vi "test-state-space-utils.vi"() -> ()   [LabVIEW 2019]
uses:
  <vilib>/Rock Robotics/WPI/ThirdParty/JAS_Junk/TrajLib/LINEAR_SYSTEM.ctl
  <vilib>/Analysis/Matrix/Datatypes/RealMatrix.ctl
  <vilib>/Rock Robotics/WPI/ThirdParty/JAS_Junk/TrajLib/LINEAR_QUADRATIC_REGULATOR.ctl
  <vilib>/Rock Robotics/WPI/ThirdParty/JAS_Junk/TrajLib/DCMotor_New.vi
  <vilib>/Rock Robotics/WPI/ThirdParty/JAS_Junk/TrajLib/Units_RotationsPerMinuteToRadiansPerSecond.vi
  <vilib>/Rock Robotics/WPI/ThirdParty/JAS_Junk/TrajLib/LinearSystem_New.vi
  <vilib>/Rock Robotics/WPI/ThirdParty/JAS_Junk/TrajLib/MatBuilder_Create.vi
  <vilib>/Rock Robotics/WPI/ThirdParty/JAS_Junk/TrajLib/MatBuilder_Fill.vi
  <vilib>/Rock Robotics/WPI/ThirdParty/JAS_Junk/TrajLib/MatrixHelper_Zero.vi
  <vilib>/Rock Robotics/WPI/ThirdParty/JAS_Junk/TrajLib/MatrixHelper_CoerceSize.vi
  <vilib>/Rock Robotics/WPI/ThirdParty/JAS_Junk/TrajLib/Trajectory_Library.lvlib
  <vilib>/Analysis/Matrix/NI_Matrix.lvlib
panel:
  out "LQR New Sys-ELMS Error":bool
  out "LQR New Error":bool
  out "LQR New":T1
  out "Rcost":T2
  out "Qcost":T2
  out "Relms":T2
  out "Qelms":T2
  out "LQR New Sys-ELMS":T1
  out "ElevatorSystem":T3
  # "Ref State <States,1>"
  # "Comp and capped \noutput <Inputs,1>"
  # "Controller gain\n<Inputs,States>"
  # "Ref State <States,1>"
  # "Comp and capped \noutput <Inputs,1>"
  # "Controller gain\n<Inputs,States>"
  # "<States,States>"
  # "<States,Inputs>"
  # "<Outputs,States>"
  # "<Outputs,Inputs>"
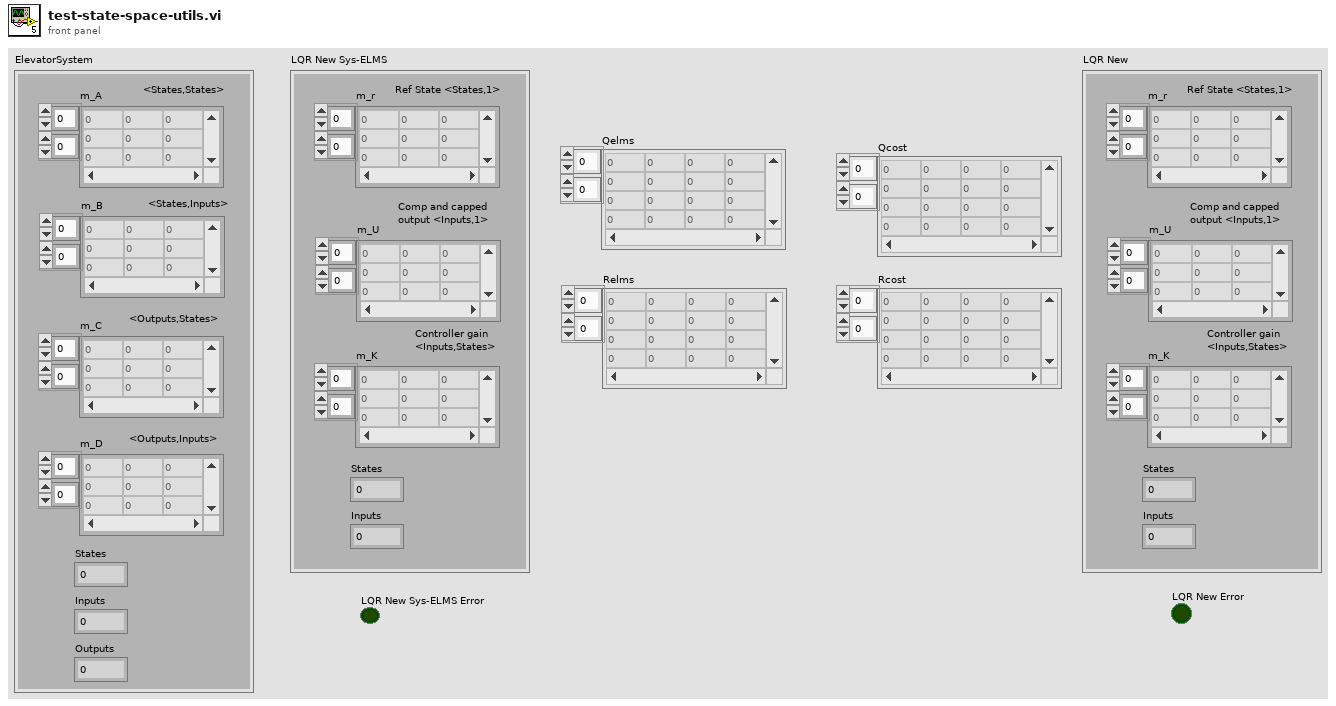
[diagram p1: front panel]
types:
  T1 = typedef "Trajectory_Library.lvlib/LINEAR_QUADRATIC_REGULATOR.ctl" = cluster{"m_r":T2, "m_U":T2, "m_K":T2, "States":i32, "Inputs":i32}
  T2 = typedef "NI_Matrix.lvlib/RealMatrix.ctl" = dbl[][]
  T3 = typedef "Trajectory_Library.lvlib/LINEAR_SYSTEM.ctl" = cluster{"m_A":T2, "m_B":T2, "m_C":T2, "m_D":T2, "States":i32, "Inputs":i32, "Outputs":i32}
  T4 = typedef "Trajectory_Library.lvlib/DCMOTOR.CTL" = cluster{"nominalVoltage_Volts":dbl, "StallTorque_NM":dbl, "StallCurrent_Amps":dbl, "FreeCurrent_Amps":dbl, "FreeSpeed_RadPerSec":dbl, "R_Ohms":dbl, "Kv_RadPerSecPerVolt":dbl, "Kt_NMPerAmp":dbl}
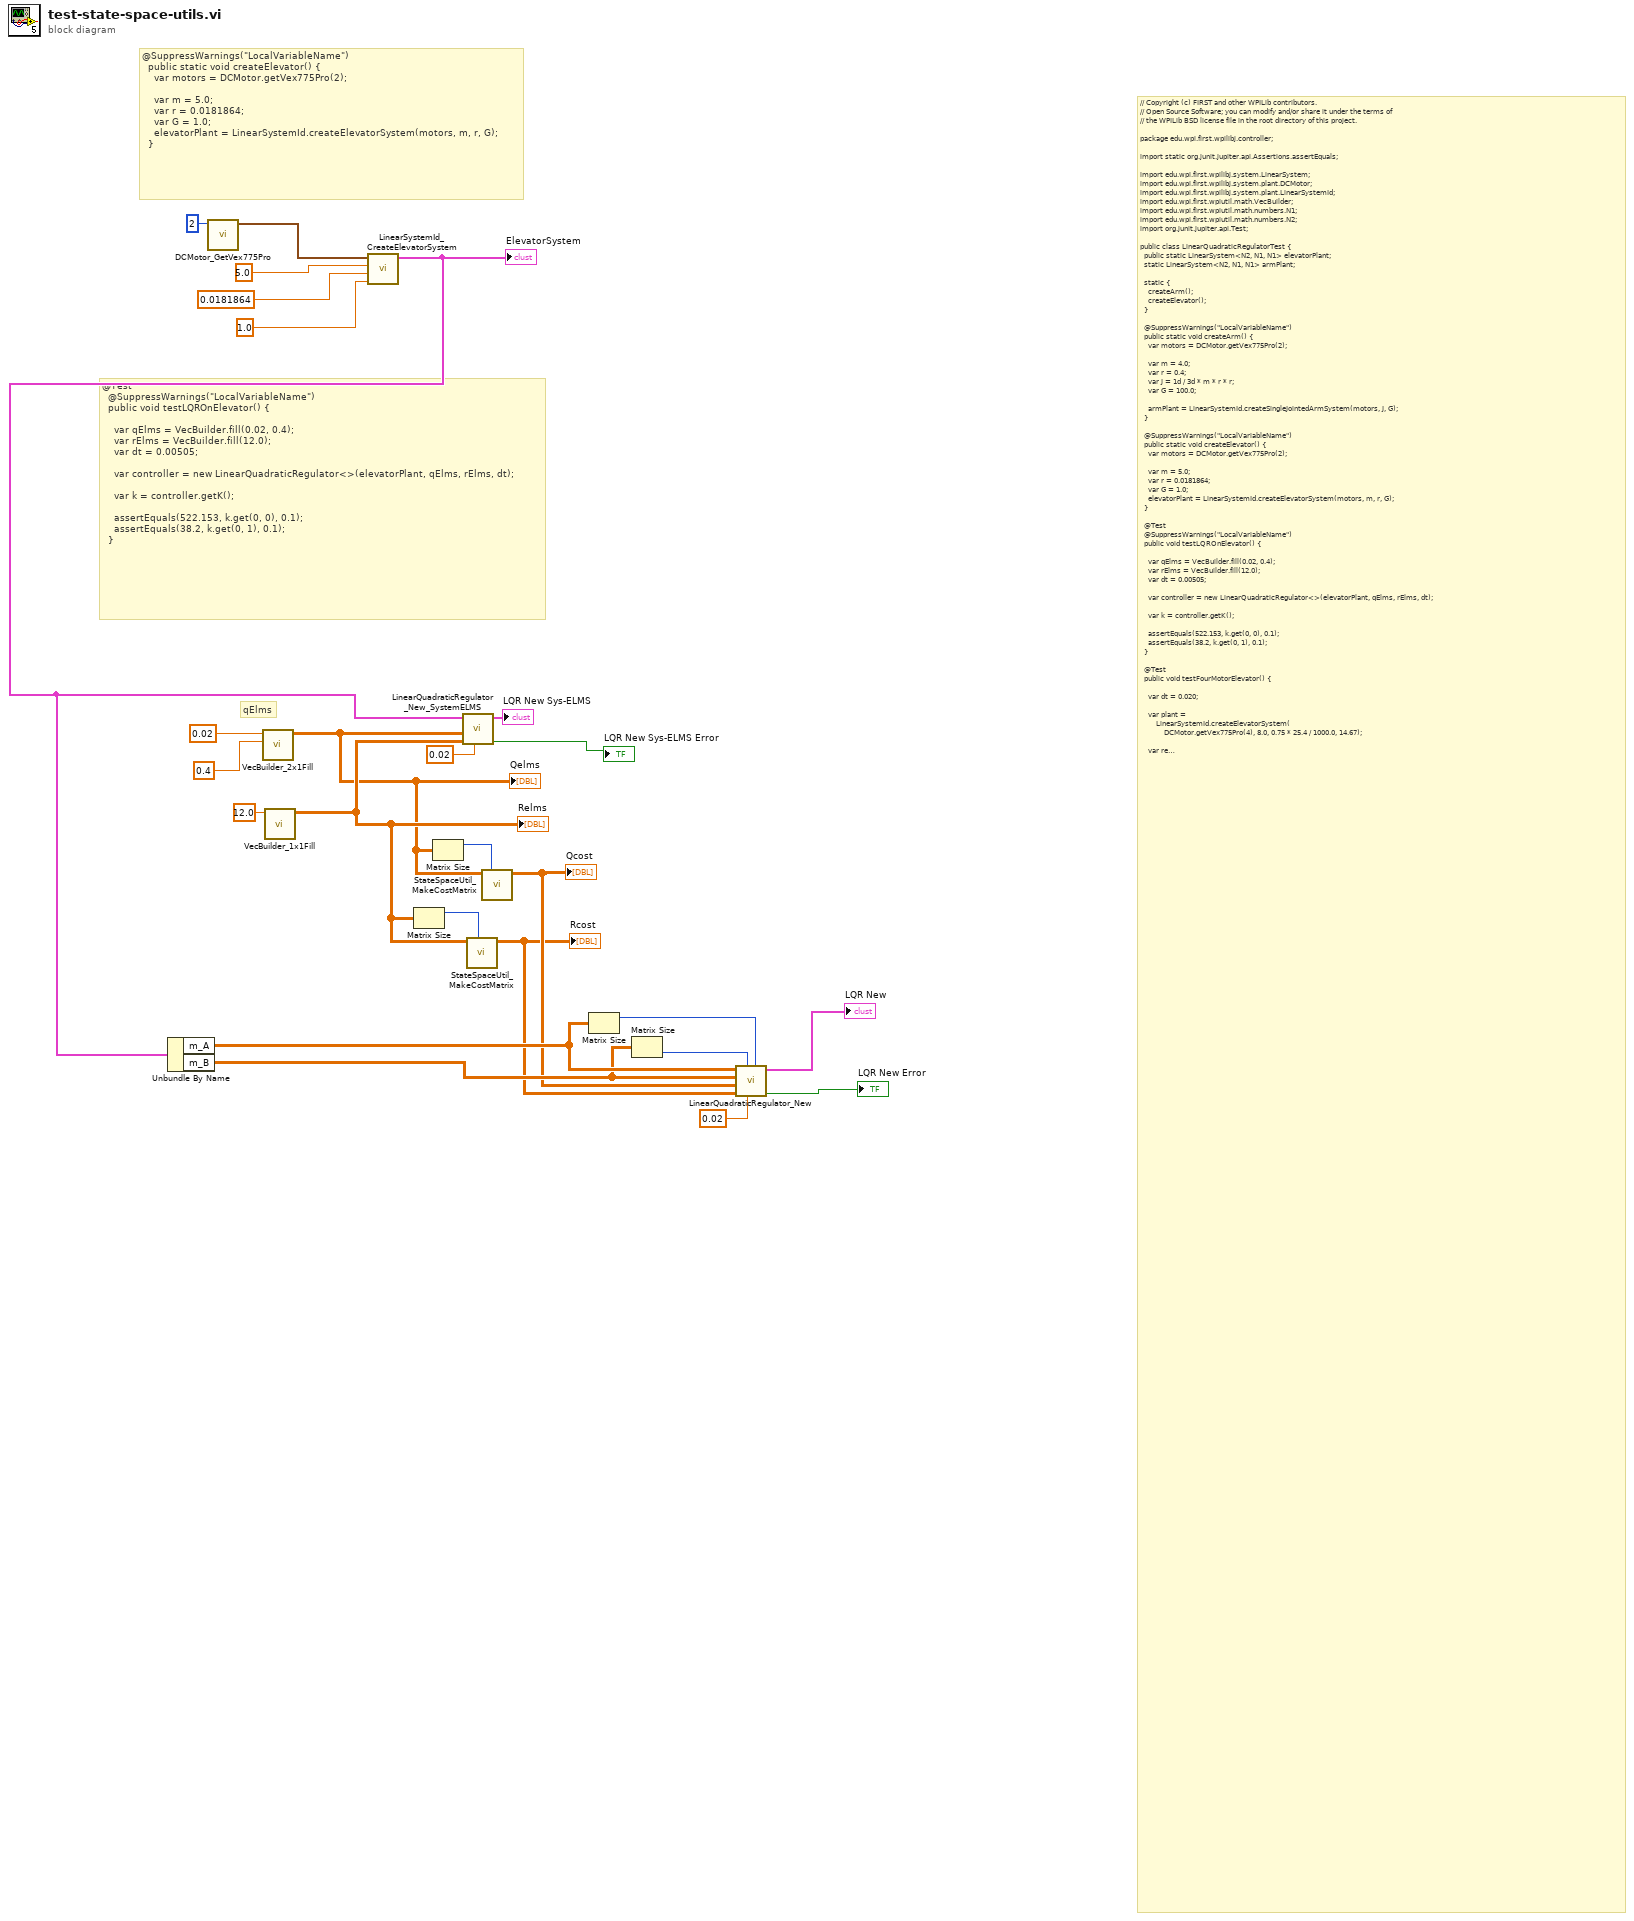
[diagram p0: block diagram]
diagram:
  # "@SuppressWarnings(\"LocalVariableName\")\n  public static void createElevator() {\n    var motors = DCMotor.getVex775Pro(2);\n\n    var m = 5.0;\n    var r = 0.0181864;\n    var G = 1.0;\n    elevatorPlant = LinearSystemId.createElevatorSystem(motors, m, r, G);\n  }"
  # "qElms"
  # "@Test\n  @SuppressWarnings(\"LocalVariableName\")\n  public void testLQROnElevator() {\n\n    var qElms = VecBuilder.fill(0.02, 0.4);\n    var rElms = VecBuilder.fill(12.0);\n    var dt = 0.00505;\n\n    var controller = new LinearQuadraticRegulator<>(elevatorPlant, qElms, rElms, dt);\n\n    var k = controller.getK();\n\n    assertEquals(522.153, k.get(0, 0), 0.1);\n    assertEquals(38.2, k.get(0, 1), 0.1);\n  }"
  # "// Copyright (c) FIRST and other WPILib contributors.\n// Open Source Software; you can modify and/or share it under the terms of\n// the WPILib BSD license file in the root directory of this project.\n\npackage edu.wpi.first.wpilibj.controller;\n\nimport static org.junit.jupiter.api.Assertions.assertEquals;\n\nimport edu.wpi.first.wpilibj.system.LinearSystem;\nimport edu.wpi.first.wpilibj.system.plant.DCMotor;\nimport edu.wpi.first.wpilibj.system.plant.LinearSystemId;\nimport edu.wpi.first.wpiutil.math.VecBuilder;\nimport edu.wpi.first.wpiutil.math.numbers.N1;\nimport edu.wpi.first.wpiutil.math.numbers.N2;\nimport org.junit.jupiter.api.Test;\n\npublic class LinearQuadraticRegulatorTest {\n  public static LinearSystem<N2, N1, N1> elevatorPlant;\n  static LinearSystem<N2, N1, N1> armPlant;\n\n  static {\n    createArm();\n    createElevator();\n  }\n\n  @SuppressWarnings(\"LocalVariableName\")\n  public static void createArm() {\n    var motors = DCMotor.getVex775Pro(2);\n\n    var m = 4.0;\n    var r = 0.4;\n    var J = 1d / 3d * m * r * r;\n    var G = 100.0;\n\n    armPlant = LinearSystemId.createSingleJointedArmSystem(motors, J, G);\n  }\n\n  @SuppressWarnings(\"LocalVariableName\")\n  public static void createElevator() {\n    var motors = DCMotor.getVex775Pro(2);\n\n    var m = 5.0;\n    var r = 0.0181864;\n    var G = 1.0;\n    elevatorPlant = LinearSystemId.createElevatorSystem(motors, m, r, G);\n  }\n\n  @Test\n  @SuppressWarnings(\"LocalVariableName\")\n  public void testLQROnElevator() {\n\n    var qElms = VecBuilder.fill(0.02, 0.4);\n    var rElms = VecBuilder.fill(12.0);\n    var dt = 0.00505;\n\n    var controller = new LinearQuadraticRegulator<>(elevatorPlant, qElms, rElms, dt);\n\n    var k = controller.getK();\n\n    assertEquals(522.153, k.get(0, 0), 0.1);\n    assertEquals(38.2, k.get(0, 1), 0.1);\n  }\n\n  @Test\n  public void testFourMotorElevator() {\n\n    var dt = 0.020;\n\n    var plant =\n        LinearSystemId.createElevatorSystem(\n            DCMotor.getVex775Pro(4), 8.0, 0.75 * 25.4 / 1000.0, 14.67);\n\n    var regulator =\n        new LinearQuadraticRegulator<>(plant, VecBuilder.fill(0.1, 0.2), VecBuilder.fill(12.0), dt);\n\n    assertEquals(10.381, regulator.getK().get(0, 0), 1e-2);\n    assertEquals(0.6929, regulator.getK().get(0, 1), 1e-2);\n  }\n\n  @Test\n  @SuppressWarnings(\"LocalVariableName\")\n  public void testLQROnArm() {\n\n    var motors = DCMotor.getVex775Pro(2);\n\n    var m = 4.0;\n    var r = 0.4;\n    var G = 100.0;\n\n    var plant = LinearSystemId.createSingleJointedArmSystem(motors, 1d / 3d * m * r * r, G);\n\n    var qElms = VecBuilder.fill(0.01745, 0.08726);\n    var rElms = VecBuilder.fill(12.0);\n    var dt = 0.00505;\n\n    var controller = new LinearQuadraticRegulator<>(plant, qElms, rElms, dt);\n\n    var k = controller.getK();\n\n    assertEquals(19.16, k.get(0, 0), 0.1);\n    assertEquals(3.32, k.get(0, 1), 0.1);\n  }\n\n  @Test\n  public void testLatencyCompensate() {\n    var dt = 0.02;\n\n    var plant =\n        LinearSystemId.createElevatorSystem(\n            DCMotor.getVex775Pro(4), 8.0, 0.75 * 25.4 / 1000.0, 14.67);\n\n    var regulator =\n        new LinearQuadraticRegulator<>(plant, VecBuilder.fill(0.1, 0.2), VecBuilder.fill(12.0), dt);\n\n    regulator.latencyCompensate(plant, dt, 0.01);\n\n    assertEquals(8.97115941, regulator.getK().get(0, 0), 1e-3);\n    assertEquals(0.07904881, regulator.getK().get(0, 1), 1e-3);\n  }\n}"
  n1 = call <vilib>:"DCMotor_GetVex775Pro.vi"("Num Motors"=2) -> ("DCMOTOR"=w21:T4)  [unwired: 10 in]
  n2 = call <vilib>:"VecBuilder_2x1Fill.vi"("R1"=0.4, "R0"=0.02) -> ("output matrix"=w13:T2)  [unwired: 9 in]
  "Qelms" <- w13
  n3 = call <vilib>:"VecBuilder_1x1Fill.vi"("R0_C0"=12.0) -> ("output matrix"=w15:T2)  [unwired: 10 in]
  "Relms" <- w15
  n4 = call <vilib>:"LinearSystemId_CreateElevatorSystem.vi"("G"=1.0, "radiusMeters"=0.0181864, "massKg"=5.0, "DCMOTOR"=w21) -> ("Linearsystem"=w11:T3)  [unwired: 7 in]
  "ElevatorSystem" <- w11
  n5 = Unbundle By Name(w11) -> ("m_A"=w10:T2, "m_B"=w8:T2)
  n6 = Matrix Size(0:w15) -> (1:w14:i32)  [unwired: 1 out]
  n7 = Matrix Size(0:w13) -> (1:w12:i32)  [unwired: 1 out]
  n8 = call <vilib>:"LinearQuadraticRegulator_New_SystemELMS.vi"("dt_Seconds"=0.02, "Relms"=w15, "Qelms"=w13, "LINEARSYSTEM"=w11) -> ("Error"=→"LQR New Sys-ELMS Error":bool, "LinearQuadraticRegulator"=→"LQR New Sys-ELMS":T1)  [unwired: 6 in]
  n9 = call <vilib>:"StateSpaceUtil_MakeCostMatrix.vi"("States"=w14, "Costs"=w15) -> ("Costs Matrix"=w5:T2)  [unwired: 9 in]
  "Rcost" <- w5
  n10 = call <vilib>:"StateSpaceUtil_MakeCostMatrix.vi"("States"=w12, "Costs"=w13) -> ("Costs Matrix"=w6:T2)  [unwired: 9 in]
  "Qcost" <- w6
  n11 = Matrix Size(0:w10) -> (1:w9:i32)  [unwired: 1 out]
  n12 = Matrix Size(0:w8) -> (2:w7:i32)  [unwired: 1 out]
  n13 = call <vilib>:"LinearQuadraticRegulator_New.vi"("States"=w9, "dt_Seconds"=0.02, "Inputs"=w7, "R"=w5, "Q"=w6, "B"=w8, "A"=w10) -> ("Error"=→"LQR New Error":bool, "LinearQuadraticRegulator"=→"LQR New":T1)  [unwired: 3 in]
